vi "Read # of Obs.vi"(8 "error in (no error)":errorcluster, 11 "Stability Step in":refnum<class "Stability Step.lvclass">) -> (0 "error out":errorcluster, 2 "# of Obs":u16, 3 "Stability Step out":refnum<class "Stability Step.lvclass">)   [LabVIEW 2015, in "Stability Step.lvclass"]
uses:
  Stability Step.lvclass
  Stability Step.lvclass/Stability Step.ctl
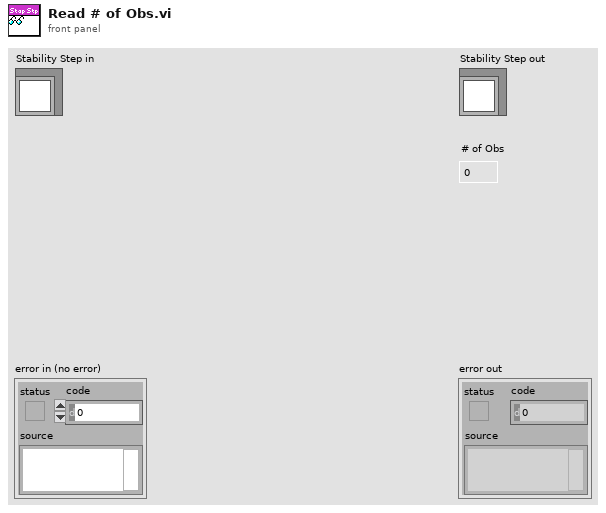
[diagram p1: front panel]
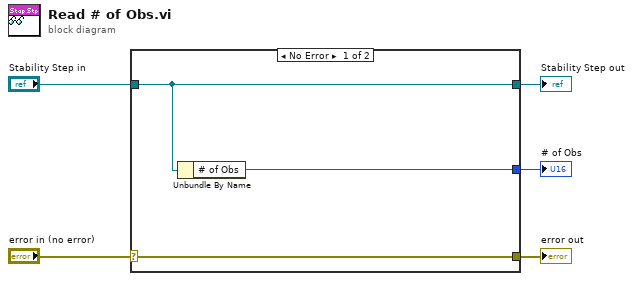
[diagram p0: block diagram]
diagram:
  n1 = case shown="No Error" "error in (no error)" {
    selector: "error in (no error)" -> [w8 w9]
    tunnel: [w8 w9] -> w4
    tunnel: [w7 w10] -> w2
    tunnel: "Stability Step in" -> [w7 w10]
    tunnel: [w6 _] -> w1
    frame No Error {
      n2 = Unbundle By Name(w7) -> ("# of Obs"=w6:u16)
    }
    frame Error {
    }
  }
  "error out" <- w4
  "Stability Step out" <- w2
  "# of Obs" <- w1
